vi "TableDataToGraph.vi"(0 "Data Table":dbl[][](array[numeric])) -> (1 "Speed Graph":cluster{dbl[], "Data Table":dbl[]}[](array[cluster]), 2 "Pressure Graph":cluster{dbl[], "Data Table":dbl[]}[](array[cluster]))   [LabVIEW 2024]
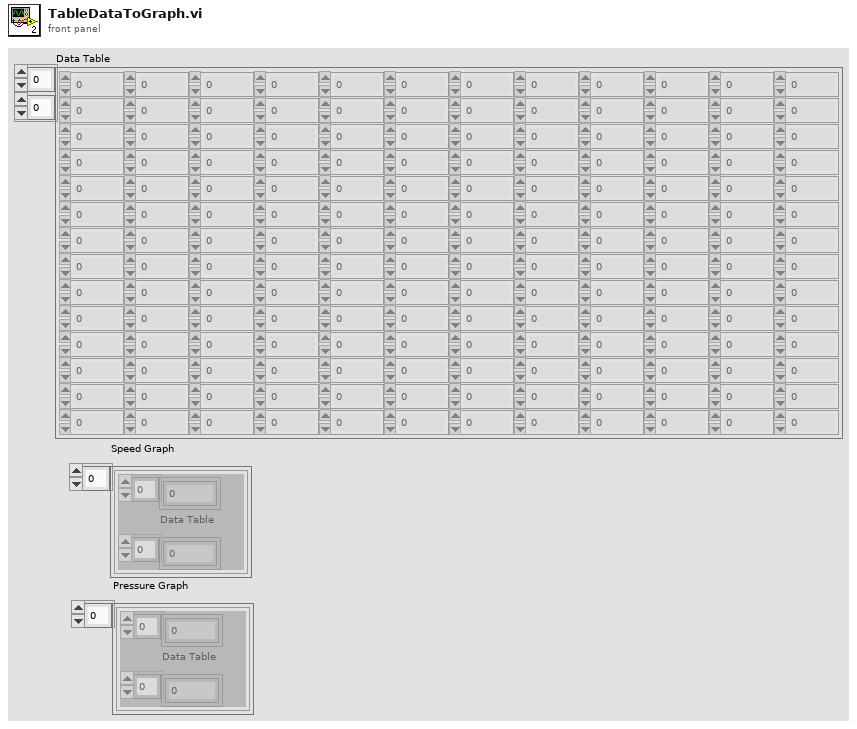
[diagram p1: front panel]
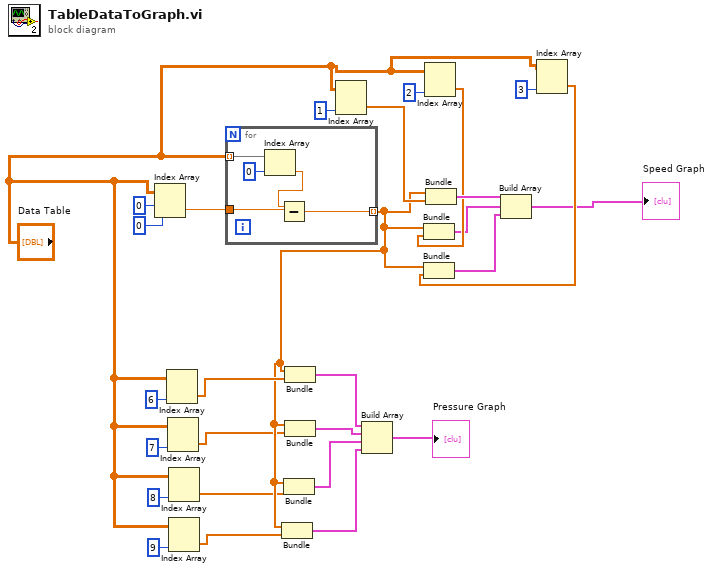
[diagram p0: block diagram]
diagram:
  n1 = Index Array(array="Data Table", index (row)=0, index (col)=0 ("disabled index (col)")) -> (element=w26:dbl)
  n2 = Index Array(array="Data Table", index (col)=6 ("disabled index (col)")) -> (element=w10:dbl[])  [unwired: 1 in]
  n3 = Index Array(array="Data Table", index (col)=7 ("disabled index (col)")) -> (element=w8:dbl[])  [unwired: 1 in]
  n4 = Index Array(array="Data Table", index (col)=8 ("disabled index (col)")) -> (element=w7:dbl[])  [unwired: 1 in]
  n5 = Index Array(array="Data Table", index (col)=9 ("disabled index (col)")) -> (element=w6:dbl[])  [unwired: 1 in]
  n6 = for {
    tunnel: "Data Table" -> [w30] mode=indexing
    tunnel: w26 -> [w31]
    tunnel: [w29] -> w9 mode=indexing
    n7 = Index Array(array=w30, index=0) -> (element=w32:dbl)
    n8 = Subtract(x=w32, y=w31) -> (x-y=w29:dbl)
  }
  n9 = Bundle(w9, "Data Table"=w6) -> (w2:cluster{dbl[], "Data Table":dbl[]})  [unwired: 1 in]
  n10 = Bundle(w9, "Data Table"=w7) -> (w3:cluster{dbl[], "Data Table":dbl[]})  [unwired: 1 in]
  n11 = Bundle(w9, "Data Table"=w10) -> (w5:cluster{dbl[], "Data Table":dbl[]})  [unwired: 1 in]
  n12 = Bundle(w9, "Data Table"=w8) -> (w4:cluster{dbl[], "Data Table":dbl[]})  [unwired: 1 in]
  n13 = Index Array(array="Data Table", index (col)=1 ("disabled index (col)")) -> (element=w23:dbl[])  [unwired: 1 in]
  n14 = Build Array(w5, w4, w3, w2) -> (→"Pressure Graph":cluster{dbl[], "Data Table":dbl[]}[])
  n15 = Index Array(array="Data Table", index (col)=2 ("disabled index (col)")) -> (element=w20:dbl[])  [unwired: 1 in]
  n16 = Bundle(w9, "Data Table"=w20) -> (w18:cluster{dbl[], "Data Table":dbl[]})  [unwired: 1 in]
  n17 = Bundle(w9, "Data Table"=w23) -> (w25:cluster{dbl[], "Data Table":dbl[]})  [unwired: 1 in]
  n18 = Index Array(array="Data Table", index (col)=3 ("disabled index (col)")) -> (element=w19:dbl[])  [unwired: 1 in]
  n19 = Bundle(w9, "Data Table"=w19) -> (w17:cluster{dbl[], "Data Table":dbl[]})  [unwired: 1 in]
  n20 = Build Array(w25, w18, w17) -> (→"Speed Graph":cluster{dbl[], "Data Table":dbl[]}[])
